vi "New Device Dialog.vi"(8 "error in":errorcluster, 11 "Config in":refnum<class "Config.lvclass">) -> (0 "error out":errorcluster, 1 "Class Path":path, 2 "Cancelled":bool, 3 "Config out":refnum<class "Config.lvclass">)   [LabVIEW 2023, in "Config.lvlib" / "Config.lvclass"]
uses:
  Config.lvclass
  Config.lvclass/Config.ctl
panel:
  in  "Cancel":bool
  in  "OK":bool caption="OK2"
  in  "Class":u16(ring)
  in  "Device":string
  # "Enter a name for the new device and select a class"
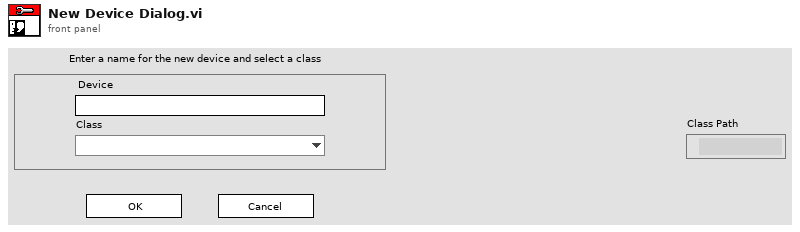
[diagram p1: front panel]
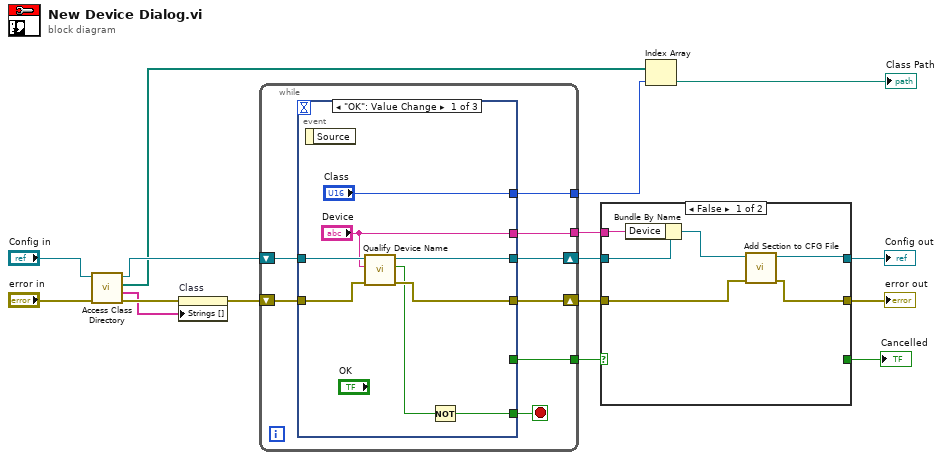
[diagram p0: block diagram]
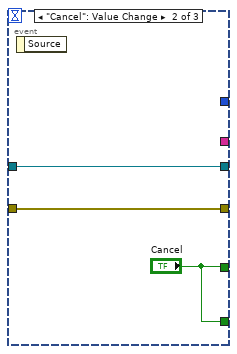
[diagram p3: hidden frame]
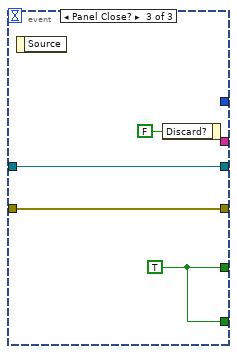
[diagram p4: hidden frame]
diagram:
  n1 = call "Access Class Directory.vi"("error in"="error in", "Config in"="Config in") -> ("error out"=w13:errorcluster, "Class Names"=w12:string[], "Class Paths"=w10:path[], "Config out"=w11:refnum<class "Config.lvclass">)  [unwired: 6 in]
  n2 = property on="Class" class="Ring (strict)"(error in=w13, "Strings []"=w12) -> (error out=w16:errorcluster)  [unwired: 1 in, 1 out]
  n3 = while {
    shift-right: [w21] -> w7
    shift-left: w11 -> [w20]
    shift-right: [w22] -> w5
    shift-left: w16 -> [w23]
    tunnel: [w19] -> w8
    tunnel: [w18] -> w3
    tunnel: [w17] -> w1
    stop <- w24 stop-if-true
    n4 = event shown="[0] \"OK\": Value Change" {
      selector: _ -> [_ _ _]
      dyn-events: _ -> [_ _ _]
      timeout: _ -> [_ _ _]
      tunnel: [w26 "Cancel" w36] -> w24
      tunnel: w23 -> [w30 w35 w38]
      tunnel: [w29 w35 w38] -> w22
      tunnel: [w31 w34 w39] -> w21
      tunnel: w20 -> [w32 w34 w39]
      tunnel: [_ "Cancel" w36] -> w18
      tunnel: ["Class" _ _] -> w19
      tunnel: ["Device" _ _] -> w17
      event "OK": Value Change {
        n5 = event-data() -> ()  [unwired: 1 in, 1 out]
        n6 = call "Qualify Device Name.vi"("error in"=w30, "Device"="Device", "Config in"=w32) -> ("error out"=w29:errorcluster, "Illegal Name"=w28:bool, "Config out"=w31:refnum<class "Config.lvclass">)  [unwired: 6 in]
        n7 = Not(x=w28) -> (.not. x?=w26:bool)
      }
      event "Cancel": Value Change {
        n8 = event-data() -> ()  [unwired: 1 in, 1 out]
      }
      event Panel Close? {
        w36 = TRUE ("Cancel")
        n9 = event-data() -> ()  [unwired: 1 in, 1 out]
        n10 = event-data("Discard?"=FALSE) -> ()  [unwired: 1 in, 1 out]
      }
    }
  }
  n11 = case shown="False" w3 {
    selector: w3 -> [_ w46]
    tunnel: w7 -> [w44 w48]
    tunnel: [w45 w48] -> w6
    tunnel: w5 -> [w41 w47]
    tunnel: [w42 w47] -> w4
    tunnel: [_ w46] -> w2
    tunnel: w1 -> [w40 _]
    frame False {
      n12 = Bundle By Name(cluster=w44, "Device"=w40) -> (w43:refnum<class "Config.lvclass">)
      n13 = call "Add Section to CFG File.vi"("error in"=w41, "Config in"=w43) -> ("error out"=w42:errorcluster, "Config out"=w45:refnum<class "Config.lvclass">)  [unwired: 8 in]
    }
    frame True {
    }
  }
  "error out" <- w4
  "Config out" <- w6
  "Cancelled" <- w2
  n14 = Index Array(array=w10, index=w8) -> (element=→"Class Path":path)
